vi "Construct Event Transport.vi"(10 "Event Priority (normal)":T1=enum."normal priority") -> (0 "error out":errorcluster, 2 "Tranport Event":refnum<user-event>, 3 "EventTransport":refnum<class "EventTransport.lvclass">)   [LabVIEW 2020, in "EventTransport.lvclass"]
doc: "构建事件传输"
uses:
  EventTransport.lvclass
  <vilib>/event_ctls.llb/usereventprio.ctl
  EventTransport.lvclass/EventTransport.ctl
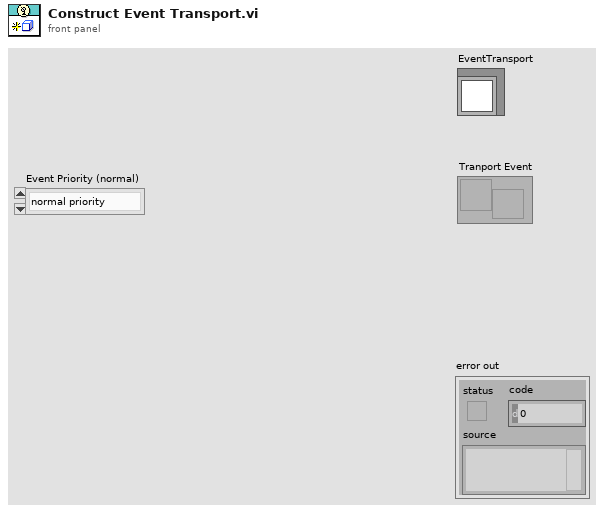
[diagram p1: front panel]
types:
  T1 = typedef "usereventprio.ctl" = enum32{"high priority", "normal priority"}
  T2 = cluster{"Data":variant, "Publication Time":timestamp}
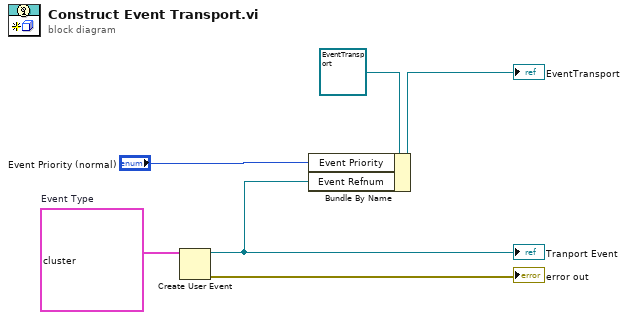
[diagram p0: block diagram]
diagram:
  w5 = T2 {"Data"=variant, "Publication Time"=timestamp(0 s since 1904-01-01)}  # Event Type
  n1 = Create User Event(user event datatype=w5) -> (user event=w3:refnum<user-event>, error out=→"error out":errorcluster)  [unwired: 1 in]
  "Tranport Event" <- w3
  n2 = Bundle By Name(cluster=refnum<class "EventTransport.lvclass"> refnum ("EventTransport"), "Event Priority"="Event Priority (normal)", "Event Refnum"=w3) -> (→"EventTransport":refnum<class "EventTransport.lvclass">)
